vi "Handle Error.vi"(7 "Stop on Unhandled Error (T)":bool=TRUE, 8 "error in":errorcluster, 11 "CircularBuffer":refnum<class "CircularBuffer.lvclass">) -> (0 "handling error":errorcluster, 2 "Unhandled error":errorcluster, 3 "CircularBuffer out":refnum<class "CircularBuffer.lvclass">)   [LabVIEW 2013, in "CircularBuffer.lvclass"]
doc: "JKI State Machine Objects (SMO) 1.0.0.11\nJKI - JKI\nCopyright (c) 2016, JKIJKI State Machine Objects (SMO) 1.0.2.13\nJKI - JKI\nCopyright (c) 2016, JKI"
uses:
  CircularBuffer.lvclass
  <vilib>/JKI/JKI SMO/SMO/SMO.lvclass
panel:
  # "For instructions on how to use the JKI State Machine Objects, examples and video tutorials, visit:\nhttp://jki.net/state-machine-objects/\n\nJKI State Machine Objects™\nhttp://jki.net/state-machine-objects/\nCopyright (C) 2005-2015, JKI <info@jki.net>\nALL RIGHTS RESERVED"
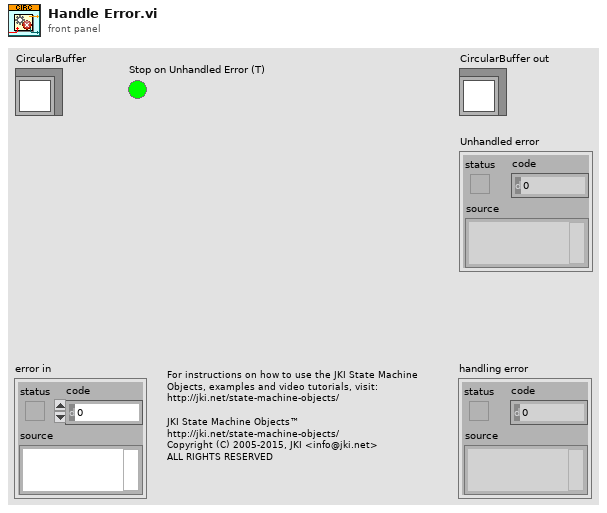
[diagram p1: front panel]
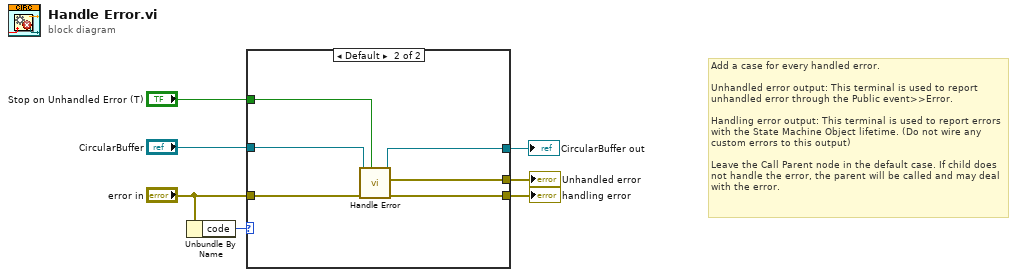
[diagram p0: block diagram]
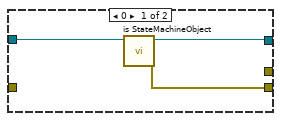
[diagram p2: hidden frame]
diagram:
  # "Add a case for every handled error.  \n\nUnhandled error output: This terminal is used to report unhandled error through the Public event>>Error.\n\nHandling error output: This terminal is used to report errors with the State Machine Object lifetime. (Do not wire any custom errors to this output)\n\nLeave the Call Parent node in the default case. If child does not handle the error, the parent will be called and may deal with the error."
  n1 = Unbundle By Name("error in") -> ("code"=w2:i32)
  n2 = case shown="Default" w2 {
    tunnel: [w8 w16] -> w7
    tunnel: [_ w15] -> w6
    tunnel: "Stop on Unhandled Error (T)" -> [_ w14]
    tunnel: "error in" -> [_ w13]
    tunnel: "CircularBuffer" -> [w10 w12]
    tunnel: [w9 w11] -> w3
    frame 0 {
      n3 = call <vilib>:"is StateMachineObject.vi"("SMO"=w10) -> ("error out"=w8:errorcluster, "SMO out"=w9:refnum<class "CircularBuffer.lvclass">)  [unwired: 8 in, 1 out]
    }
    frame Default {
      n4 = call-parent "Handle Error.vi"("Stop on Unhandled Error (T)"=w14, "error in"=w13, "SMO"=w12) -> ("handling error"=w16:errorcluster, "Unhandled error"=w15:errorcluster, "SMO out"=w11:refnum<class "CircularBuffer.lvclass">)  [unwired: 6 in]
    }
  }
  "handling error" <- w7
  "CircularBuffer out" <- w3
  "Unhandled error" <- w6
